vi "fgt set sensor Regulation Response.vi"(8 "error in (no error)":errorcluster, 10 "responseTime":u32, 11 "sensorIndex":u32) -> (0 "error out":errorcluster)   [LabVIEW 2016, in "fgt_SDK.lvlib"]
doc: "Set on a running regulation pressure response time. Minimal value is 2 for FlowEZ, 6 for MFCS controllers.\nThis function is useful if a more smooth response is wanted."
uses:
  fgt_SDK.lvlib
  dlls/fgt_SDK_32.dll
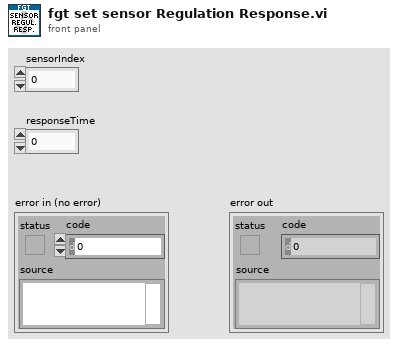
[diagram p1: front panel]
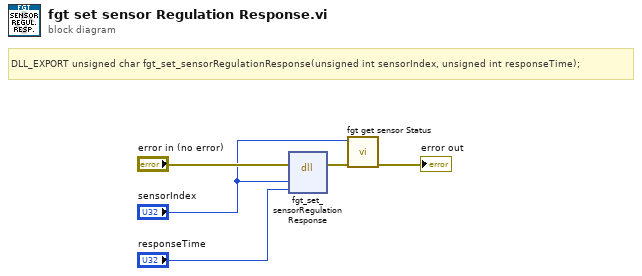
[diagram p0: block diagram]
diagram:
  # "DLL_EXPORT unsigned char fgt_set_sensorRegulationResponse(unsigned int sensorIndex, unsigned int responseTime);"
  n1 = dll-call lib="PTH2Zabs D\nMes DocumentsDéveloppementFluigentSDKsfgt-sdk-labviewdllsfgt_SDK_*.*" fn="fgt_set_sensorRegulationResponse"(error in="error in (no error)", "sensorIndex"="sensorIndex", "responseTime"="responseTime") -> (error out=w3:errorcluster)  [unwired: 5 in, 1 out]
  n2 = call "fgt get sensor Status.vi"("error in (no error)"=w3, "pressureIndex"="sensorIndex") -> ("error out"=→"error out":errorcluster)  [unwired: 9 in]
